vi "版本号读取.vi"(8 "Error in":errorcluster caption="Error in (no error)") -> (0 "error out":errorcluster, 3 "固件版本号":string)   [LabVIEW 2016, in "挥发酚.lvlib"]
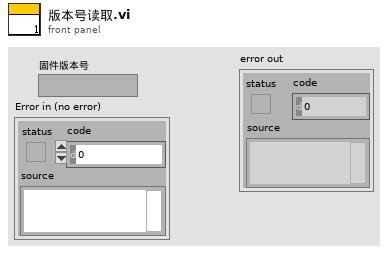
[diagram p1: front panel]
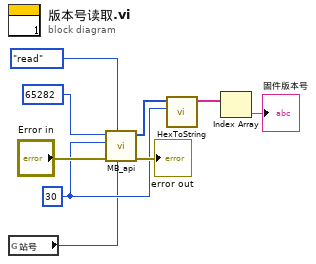
[diagram p0: block diagram]
diagram:
  w2 = u16 30 ("quantity")
  n1 = global read "挥发酚断电保存全局变量.vi" "站号"() -> (w1:u16)
  n2 = call "MB_api.vi"("Slave ID"=w1, "STEP"=enum16{"open", "read", "write", "close"}."read", "Error in"="Error in", "quantity"=w2, "starting address"=u16 65282) -> ("error out"=→"error out":errorcluster, "Registers"=w5:u16[])  [unwired: 4 in, 1 out]
  n3 = call "HexToString.vi"("字符个数"=w2, "数组"=w5) -> ("STRING"=w4:string[])  [unwired: 9 in]
  n4 = Index Array(array=w4) -> (element=→"固件版本号":string)  [unwired: 1 in]
